vi "set_wavelength.vi"(2 "error in (no error)":errorcluster, 3 "Wavelength":i32, 4 "Monochromator":refnum<visa-resource-name>="COM5") -> (0 "error":T1, 1 "Monochromator OK":bool)   [LabVIEW 2014]
uses:
  <vilib>/Instr/_visa.llb/VISA Configure Serial Port (Instr).vi
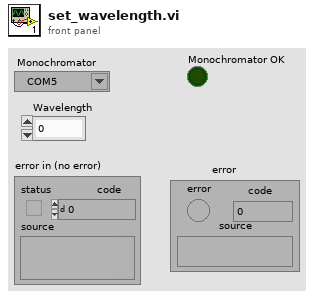
[diagram p1: front panel]
types:
  T1 = cluster{"error":bool, "code":i32, "source":string}
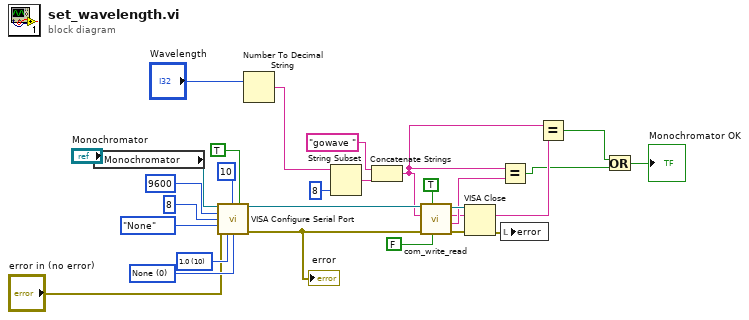
[diagram p0: block diagram]
diagram:
  w17 = u16 0 items=["None", "XON/XOFF", "RTS/CTS", "XON/XOFF & RTS/CTS", "DTR/DSR", "XON/XOFF & DTR/DSR"] ("flow control (0:none)")
  w18 = u16 10 items=["1.0"=10, "1.5"=15, "2.0"=20] ("stop bits (10: 1 bit)")
  n1 = local read "Monochromator"() -> (w22:refnum<visa-resource-name>)
  n2 = call-poly "VISA Configure Serial Port"("VISA resource name"=w22, "termination char\n(0xA = '\\n' = LF)"=u8 10 ("termination char\n(0xA = '\\n' = LF)"), "Enable Termination\nChar (T)"=TRUE, "baud rate (9600)"=u32 9600, "data bits (8)"=u16 8, "parity (0:none)"=enum16{"None", "Odd", "Even", "Mark", "Space"}."None", "error in (no error)"="error in (no error)", "stop bits (10: 1 bit)"=w18, "flow control (0:none)"=w17) -> ("VISA resource name out"=w25:refnum<visa-resource-name>, "error out"=w5:errorcluster)  [unwired: 5 in]
  "error" <- w5
  n3 = Number To Decimal String(number="Wavelength") -> (decimal integer string=w9:string)  [unwired: 1 in]
  n4 = String Subset(string=w9, length (rest)=8 ("length (rest)")) -> (substring=w14:string)  [unwired: 1 in]
  n5 = Concatenate Strings("gowave " ("write buffer"), w14) -> (w4:string)
  n6 = call "com_write_read.vi"("2 nd Query?"=FALSE, "Query?"=TRUE, "error in"=w5, "Command"=w4, "VISA handle in"=w25) -> ("error out"=w27:errorcluster, "2nd Response"=w7:string, "Response"=w6:string, "VISA handle out"=w26:refnum<visa-resource-name>)  [unwired: 1 in, 1 out]
  n7 = VISA Close(VISA resource name=w26, error in (no error)=w27) -> (error out=w23:errorcluster)
  n8 = Equal?(x=w4, y=w7) -> (x = y?=w3:bool)
  n9 = local write "error"(w23) -> ()
  n10 = Equal?(x=w4, y=w6) -> (x = y?=w2:bool)
  n11 = Or(x=w2, y=w3) -> (x .or. y?=→"Monochromator OK":bool)
